vi "Analogue Read.vi"(8 "error in":errorcluster, 10 "sampling freq: fs":dbl=1000.0, 11 "task/channels in":refnum<k21>) -> (0 "error out":errorcluster, 2 "Measured Tension":dbl[](array[numeric]), 3 "task out":refnum<k21>)   [LabVIEW 2021]
uses:
  <vilib>/Analysis/3filter.llb/Filter Passband Type.ctl
  <vilib>/DAQmx/read.llb/DAQmx Read (Analog 1D DBL NChan 1Samp).vi
  <vilib>/DAQmx/miscellaneous.llb/DAQmx Fill In Error Info.vi
  <vilib>/ptbypt/NI_PtbyPt.lvlib
  <vilib>/Analysis/NI_AALBase.lvlib
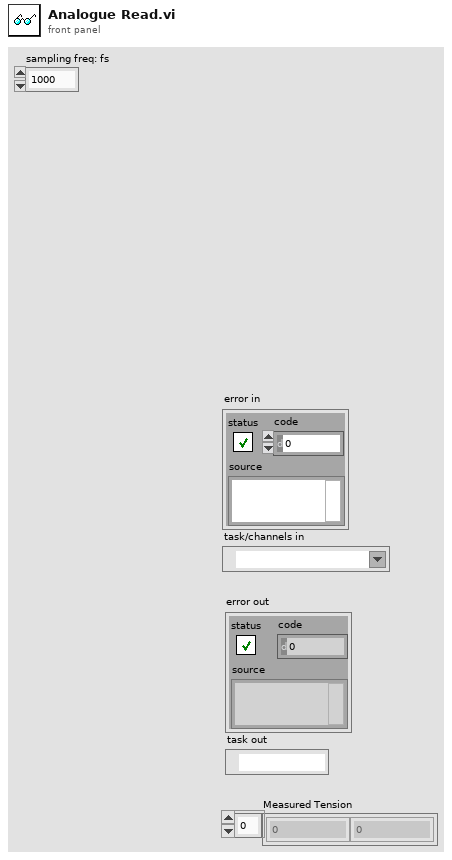
[diagram p1: front panel]
types:
  T1 = typedef "NI_AALBase.lvlib/Filter Passband Type.ctl" = enum32{"Lowpass", "Highpass", "Bandpass", "Bandstop"}
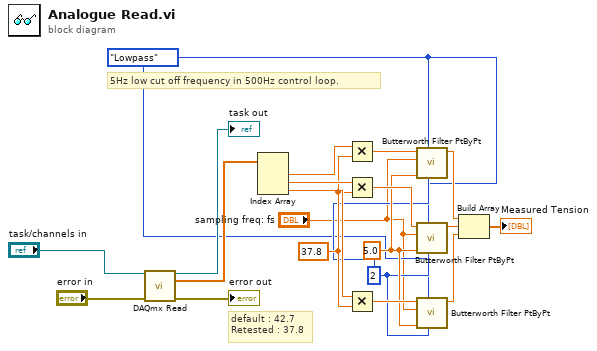
[diagram p0: block diagram]
diagram:
  w3 = 2 ("order")
  w4 = 5.0 ("low cutoff freq: fl")
  w7 = 37.8 ("y")
  w2 = Filter_Passband_Type."Lowpass" ("filter type")
  # "5Hz low cut off frequency in 500Hz control loop."
  # "default : 42.7\nRetested : 37.8"
  n1 = call-poly <vilib>:"DAQmx Read.vi"("task/channels in"="task/channels in", "error in"="error in") -> ("task out"=→"task out":refnum<k21>, "data"=w11:dbl[], "error out"=→"error out":errorcluster)  [unwired: 11 in]
  n2 = Index Array(array=w11) -> (element #1=w14:dbl, element #2=w13:dbl, element #3=w8:dbl)  [unwired: 3 in]
  n3 = Multiply(x=w14, y=w7) -> (x*y=w15:dbl)
  n4 = Multiply(x=w13, y=w7) -> (x*y=w12:dbl)
  n5 = Multiply(x=w8, y=w7) -> (x*y=w6:dbl)
  n6 = call <vilib>:"Butterworth Filter PtByPt.vi"("order"=w3, "filter type"=w2, "low cutoff freq: fl"=w4, "sampling freq: fs"="sampling freq: fs", "x"=w15) -> ("Filtered x"=w20:dbl)  [unwired: 4 in, 1 out]
  n7 = call <vilib>:"Butterworth Filter PtByPt.vi"("order"=w3, "filter type"=w2, "low cutoff freq: fl"=w4, "sampling freq: fs"="sampling freq: fs", "x"=w12) -> ("Filtered x"=w19:dbl)  [unwired: 4 in, 1 out]
  n8 = call <vilib>:"Butterworth Filter PtByPt.vi"("order"=w3, "filter type"=w2, "low cutoff freq: fl"=w4, "sampling freq: fs"="sampling freq: fs", "x"=w6) -> ("Filtered x"=w5:dbl)  [unwired: 4 in, 1 out]
  n9 = Build Array(w20, w19, w5) -> (→"Measured Tension":dbl[])
